vi "TDMS_gamepadOne.vi"(9 "POVs":i16[](array[numeric]), 10 "Buttons":bool[](array[boolean]), 11 "Axes":dbl[](array[numeric])) -> ()   [LabVIEW 2018]
uses:
  <userlib>/836-Library/System/TDMS_V2/Support/TDMS_DevRef.ctl
  <userlib>/836-Library/System/TDMS_V2/Support/Logging_Settings.ctl
  <userlib>/836-Library/System/TDMS_V2/Support/Group_FIFO_Config.ctl
  <userlib>/836-Library/System/TDMS_V2/Support/Channel_FIFO_Config.ctl
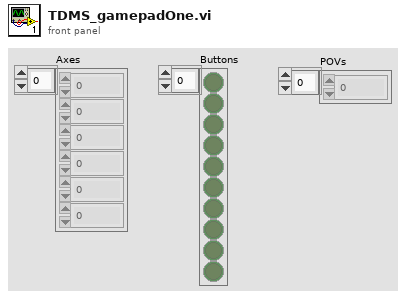
[diagram p1: front panel]
types:
  T1 = typedef "TDMS_DevRef.ctl" = cluster{"Name":string, "File Ref":refnum<k34>, "Start Time":timestamp, "Logging Settings":T2, "Group FIFO Config":T3[], "Data To Write":refnum<data-value>, "semaphore":T5, "Ref Time Reset":refnum<k4>}
  T2 = typedef "Logging_Settings.ctl" = cluster{"Data Grab Period":dbl, "File Write Period":dbl, "Max Stored Size":dbl, "Burst Size":dbl}
  T3 = typedef "Group_FIFO_Config.ctl" = cluster{"Group":string, "Channels":T4[], "Channel Names":string[]}
  T4 = typedef "Channel_FIFO_Config.ctl" = cluster{"Channel":string, "FIFO":refnum<k33>}
  T5 = typedef "Semaphore RefNum" = refnum<k1>
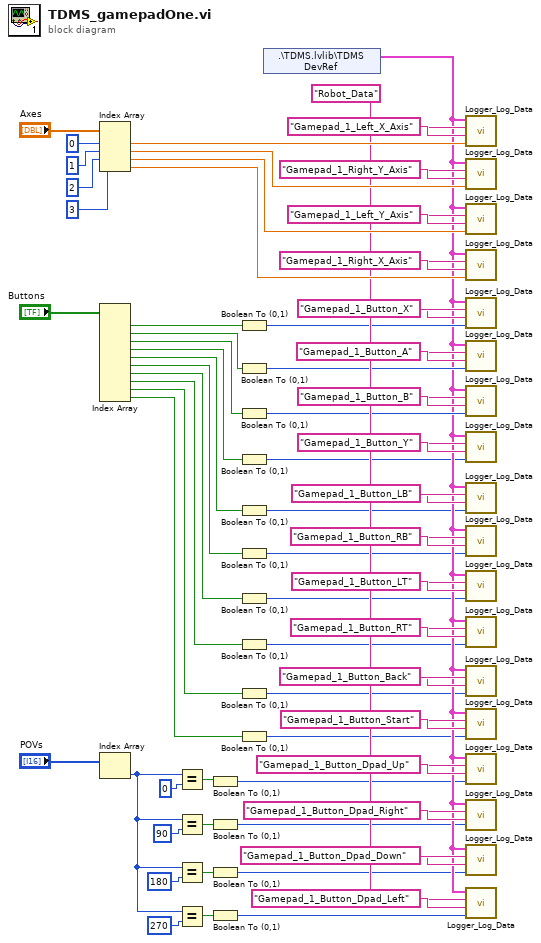
[diagram p0: block diagram]
diagram:
  w41 = "Robot_Data" ("Group")
  n1 = Index Array(array="Axes", index #1=0 ("index"), index #2=1 ("index"), index #3=2 ("index"), index #4=3 ("index")) -> (element #1=w56:dbl, element #2=w54:dbl, element #3=w53:dbl, element #4=w52:dbl)
  n2 = Index Array(array="Buttons") -> (element #1=w35:bool, element #2=w29:bool, element #3=w22:bool, element #4=w21:bool, element #5=w20:bool, element #6=w19:bool, element #7=w18:bool, element #8=w17:bool, element #9=w16:bool, element #10=w15:bool)  [unwired: 10 in]
  n3 = Index Array(array="POVs") -> (element=w10:i16)  [unwired: 1 in]
  n4 = Equal?(x=w10, y=i16 0) -> (x = y?=w9:bool)
  n5 = Equal?(x=w10, y=i16 90) -> (x = y?=w7:bool)
  n6 = Equal?(x=w10, y=i16 180) -> (x = y?=w5:bool)
  n7 = Equal?(x=w10, y=i16 270) -> (x = y?=w3:bool)
  n8 = Boolean To (0,1)(Boolean=w9) -> (0, 1=w8:i16)
  n9 = Boolean To (0,1)(Boolean=w7) -> (0, 1=w6:i16)
  n10 = Boolean To (0,1)(Boolean=w5) -> (0, 1=w4:i16)
  n11 = Boolean To (0,1)(Boolean=w3) -> (0, 1=w2:i16)
  n12 = Boolean To (0,1)(Boolean=w35) -> (0, 1=w36:i16)
  n13 = Boolean To (0,1)(Boolean=w29) -> (0, 1=w33:i16)
  n14 = Boolean To (0,1)(Boolean=w22) -> (0, 1=w32:i16)
  n15 = Boolean To (0,1)(Boolean=w21) -> (0, 1=w28:i16)
  n16 = Boolean To (0,1)(Boolean=w20) -> (0, 1=w30:i16)
  n17 = Boolean To (0,1)(Boolean=w19) -> (0, 1=w27:i16)
  n18 = Boolean To (0,1)(Boolean=w18) -> (0, 1=w26:i16)
  n19 = Boolean To (0,1)(Boolean=w17) -> (0, 1=w25:i16)
  n20 = Boolean To (0,1)(Boolean=w16) -> (0, 1=w24:i16)
  n21 = Boolean To (0,1)(Boolean=w15) -> (0, 1=w23:i16)
  n22 = shared-variable ".\\TDMS.lvlib\\TDMS DevRef"() -> (w31:T1)  [unwired: 1 in, 1 out]
  n23 = call <userlib>:"Logger_Log_Data.vi"("Data"=w56, "Channel"="Gamepad_1_Left_X_Axis", "Group"=w41, "TDMS DevRef"=w31) -> ()  [unwired: 7 in, 1 out]
  n24 = call <userlib>:"Logger_Log_Data.vi"("Data"=w54, "Channel"="Gamepad_1_Right_Y_Axis", "Group"=w41, "TDMS DevRef"=w31) -> ()  [unwired: 7 in, 1 out]
  n25 = call <userlib>:"Logger_Log_Data.vi"("Data"=w53, "Channel"="Gamepad_1_Left_Y_Axis", "Group"=w41, "TDMS DevRef"=w31) -> ()  [unwired: 7 in, 1 out]
  n26 = call <userlib>:"Logger_Log_Data.vi"("Data"=w52, "Channel"="Gamepad_1_Right_X_Axis", "Group"=w41, "TDMS DevRef"=w31) -> ()  [unwired: 7 in, 1 out]
  n27 = call <userlib>:"Logger_Log_Data.vi"("Data"=w36, "Channel"="Gamepad_1_Button_X", "Group"=w41, "TDMS DevRef"=w31) -> ()  [unwired: 7 in, 1 out]
  n28 = call <userlib>:"Logger_Log_Data.vi"("Data"=w33, "Channel"="Gamepad_1_Button_A", "Group"=w41, "TDMS DevRef"=w31) -> ()  [unwired: 7 in, 1 out]
  n29 = call <userlib>:"Logger_Log_Data.vi"("Data"=w32, "Channel"="Gamepad_1_Button_B", "Group"=w41, "TDMS DevRef"=w31) -> ()  [unwired: 7 in, 1 out]
  n30 = call <userlib>:"Logger_Log_Data.vi"("Data"=w28, "Channel"="Gamepad_1_Button_Y", "Group"=w41, "TDMS DevRef"=w31) -> ()  [unwired: 7 in, 1 out]
  n31 = call <userlib>:"Logger_Log_Data.vi"("Data"=w30, "Channel"="Gamepad_1_Button_LB", "Group"=w41, "TDMS DevRef"=w31) -> ()  [unwired: 7 in, 1 out]
  n32 = call <userlib>:"Logger_Log_Data.vi"("Data"=w27, "Channel"="Gamepad_1_Button_RB", "Group"=w41, "TDMS DevRef"=w31) -> ()  [unwired: 7 in, 1 out]
  n33 = call <userlib>:"Logger_Log_Data.vi"("Data"=w26, "Channel"="Gamepad_1_Button_LT", "Group"=w41, "TDMS DevRef"=w31) -> ()  [unwired: 7 in, 1 out]
  n34 = call <userlib>:"Logger_Log_Data.vi"("Data"=w25, "Channel"="Gamepad_1_Button_RT", "Group"=w41, "TDMS DevRef"=w31) -> ()  [unwired: 7 in, 1 out]
  n35 = call <userlib>:"Logger_Log_Data.vi"("Data"=w24, "Channel"="Gamepad_1_Button_Back", "Group"=w41, "TDMS DevRef"=w31) -> ()  [unwired: 7 in, 1 out]
  n36 = call <userlib>:"Logger_Log_Data.vi"("Data"=w23, "Channel"="Gamepad_1_Button_Start", "Group"=w41, "TDMS DevRef"=w31) -> ()  [unwired: 7 in, 1 out]
  n37 = call <userlib>:"Logger_Log_Data.vi"("Data"=w8, "Channel"="Gamepad_1_Button_Dpad_Up", "Group"=w41, "TDMS DevRef"=w31) -> ()  [unwired: 7 in, 1 out]
  n38 = call <userlib>:"Logger_Log_Data.vi"("Data"=w6, "Channel"="Gamepad_1_Button_Dpad_Right", "Group"=w41, "TDMS DevRef"=w31) -> ()  [unwired: 7 in, 1 out]
  n39 = call <userlib>:"Logger_Log_Data.vi"("Data"=w4, "Channel"="Gamepad_1_Button_Dpad_Down", "Group"=w41, "TDMS DevRef"=w31) -> ()  [unwired: 7 in, 1 out]
  n40 = call <userlib>:"Logger_Log_Data.vi"("Data"=w2, "Channel"="Gamepad_1_Button_Dpad_Left", "Group"=w41, "TDMS DevRef"=w31) -> ()  [unwired: 7 in, 1 out]
